vi "16.-Promedio Señal, Tablas, Limite, Sonido y Guardar en Archivo.vi"() -> ()   [LabVIEW 2020]
panel:
  out "Peligro":bool
  in  "Limite":dbl
  in  "stop":bool
  out "error out":errorcluster
  out "Waveform Chart":cluster{dbl, "Señal":dbl, "Limite":dbl}(graph)
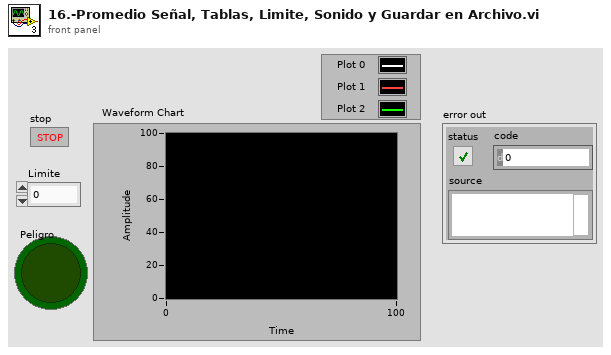
[diagram p1: front panel]
types:
  T1 = enum16{"open", "replace", "create", "open or create", "replace or create", "replace or create with confirmation"}
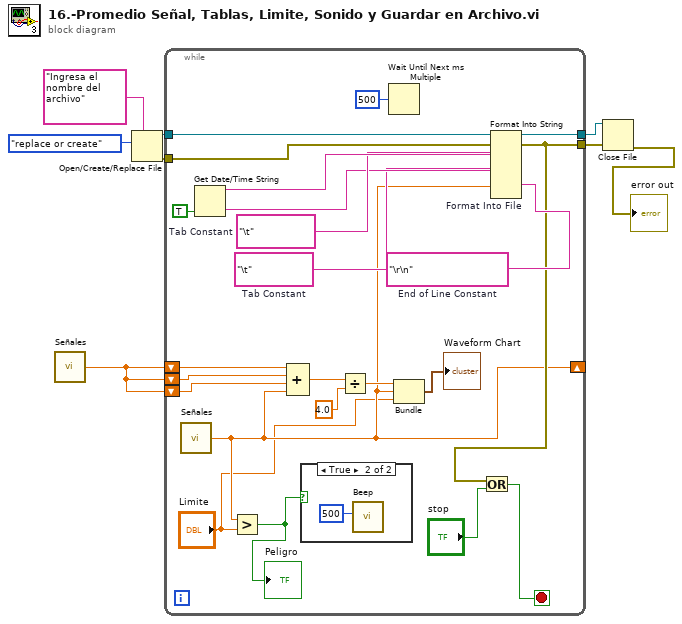
[diagram p0: block diagram]
diagram:
  n1 = call "Señales.vi"() -> ("Señal"=w4:dbl)
  n2 = Open/Create/Replace File(prompt="Ingresa el nombre del archivo", operation (0:open)=T1."replace or create") -> (refnum out=w6:refnum<file>, error out=w5:errorcluster)  [unwired: 4 in, 1 out]
  n3 = while {
    tunnel: w6 -> [w31]
    tunnel: w5 -> [w30]
    tunnel: [w29] -> w3
    tunnel: [w13] -> w2
    shift-right: [w10] -> _
    shift-left: w4 -> [w28]
    shift-left: w4 -> [w27]
    shift-left: w4 -> [w26]
    stop <- w12 stop-if-true
    w15 = "\r\n"  # End of Line Constant
    w16 = "\t"  # Tab Constant
    w18 = "\t"  # Tab Constant
    n4 = call "Señales.vi"() -> ("Señal"=w10:dbl)
    n5 = Get Date/Time String(want seconds? (F)=TRUE) -> (date string=w19:string, time string=w17:string)  [unwired: 2 in]
    n6 = Greater?(x=w10, y="Limite") -> (0:w11:bool)
    "Peligro" <- w11
    n7 = Compound Arithmetic op=ADD(w28, w27, w26, w10) -> (w25:dbl)
    n8 = case shown="True" w11 {
      frame False {
      }
      frame True {
        n9 = call <vilib>:"Beep.vi"("duration (msec)"=u32 500) -> ()  [unwired: 11 in]
      }
    }
    n10 = Divide(x=w25, y=4.0) -> (x/y=w23:dbl)
    n11 = Wait Until Next ms Multiple(millisecond multiple=u32 500) -> ()  [unwired: 1 out]
    n12 = Bundle(w23, "Señal"=w10, "Limite"="Limite") -> (→"Waveform Chart":cluster{dbl, "Señal":dbl, "Limite":dbl})  [unwired: 1 in]
    n13 = Format Into String "Format Into File"(initial string=w31, error in=w30, w19, w18, w17, w16, w10, w15) -> (resulting string=w29:refnum<file>, error out=w13:errorcluster)  [unwired: 1 in]
    n14 = Or(x=w13, y="stop") -> (x .or. y?=w12:bool)
  }
  n15 = Close File(refnum=w3, error in=w2) -> (error out=→"error out":errorcluster)  [unwired: 1 out]
